vi "Get File and Folder Details Test.vi"(8 "Error In":errorcluster) -> (0 "Error Out":errorcluster)   [LabVIEW 2023, in "Test.lvlib"]
uses:
  Test.lvlib
  <vilib>/addons/_JKI Toolkits/Caraya/classes/Assert/Assert Equal Value_Variant.vi
  <vilib>/addons/_JKI Toolkits/Caraya/classes/Test/Test.lvclass
  <vilib>/addons/_JKI Toolkits/Caraya/classes/Assert/Assert.lvclass
  File Path Operations/File and Path Operations.lvlib
panel:
  # "FILE AND FOLDER DETAILS TEST"
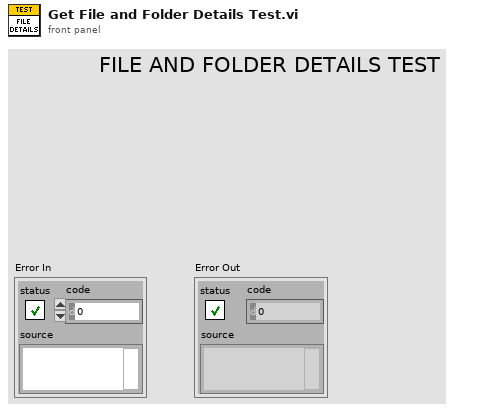
[diagram p1: front panel]
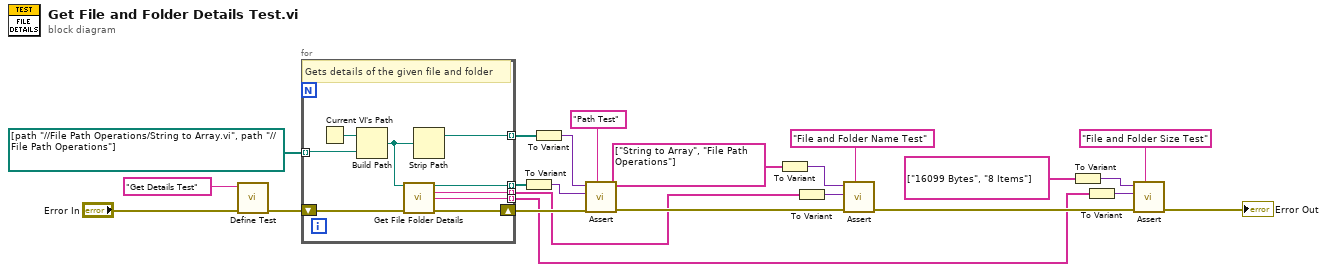
[diagram p0: block diagram]
diagram:
  n1 = call <vilib>:"Define Test.vi"("error in (no error)"="Error In", "Label (VI Title)"="Get Details Test") -> ("error out"=w21:errorcluster)  [unwired: 8 in, 1 out]
  n2 = for {
    shift-right: [w31] -> w20
    shift-left: w21 -> [w32]
    tunnel: path[] [path "../../File Path Operations/String to Array.vi", path "../../File Path Operations"] -> [w29] mode=indexing
    tunnel: [w26] -> w17 mode=indexing
    tunnel: [w24] -> w18 mode=indexing
    tunnel: [w28] -> w9 mode=indexing
    tunnel: [w27] -> w7 mode=indexing
    # "Gets details of the given file and folder"
    n3 = Current VI's Path() -> (path=w30:path)
    n4 = Build Path(base path=w30, name or relative path=w29) -> (appended path=w25:path)
    n5 = call "Get File Folder Details.vi"("Path"=w25, "Error In"=w32) -> ("Parent Path"=w26:path, "Name"=w28:string, "Size"=w27:string, "Error Out"=w31:errorcluster)  [unwired: 10 in]
    n6 = Strip Path(path=w25) -> (stripped path=w24:path)  [unwired: 1 out]
  }
  n7 = To Variant(anything=w17) -> (Variant=w15:variant)
  n8 = To Variant(anything=w18) -> (Variant=w16:variant)
  n9 = call-poly <vilib>:"Assert.vi"("Label"="Path Test", "error in (no error)"=w20, "Y"=w15, "X"=w16) -> ("error out"=w13:errorcluster)  [unwired: 6 in, 1 out]
  n10 = To Variant(anything=string[] ["String to Array", "File Path Operations"]) -> (Variant=w4:variant)
  n11 = To Variant(anything=w9) -> (Variant=w8:variant)
  n12 = call-poly <vilib>:"Assert.vi"("Label"="File and Folder Name Test", "error in (no error)"=w13, "Y"=w8, "X"=w4) -> ("error out"=w12:errorcluster)  [unwired: 6 in, 1 out]
  n13 = To Variant(anything=string[] ["16099 Bytes", "8 Items"]) -> (Variant=w1:variant)
  n14 = To Variant(anything=w7) -> (Variant=w6:variant)
  n15 = call-poly <vilib>:"Assert.vi"("Label"="File and Folder Size Test", "error in (no error)"=w12, "Y"=w6, "X"=w1) -> ("error out"=→"Error Out":errorcluster)  [unwired: 6 in, 1 out]
